vi "Query (varients).vi"(6 "timeout in ms (5000)":i32=5000, 8 "error in (no error)":errorcluster, 9 "Varient":variant, 10 "Label":string, 11 "MSR Parent":refnum<class "Send.lvclass">) -> (0 "error out":errorcluster, 1 "Replay Varient":variant, 2 "Reply Label":string, 3 "MSR Parent":refnum<class "Send.lvclass">)   [LabVIEW 2011, in "Messenging.lvlib" / "Send.lvclass"]
uses:
  Send.lvclass
  VarMessage/VarMessage.lvclass
  TextVarientMessage/MSG.lvclass
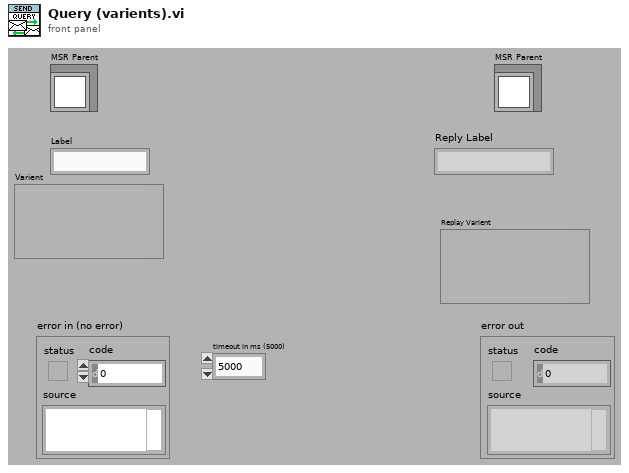
[diagram p1: front panel]
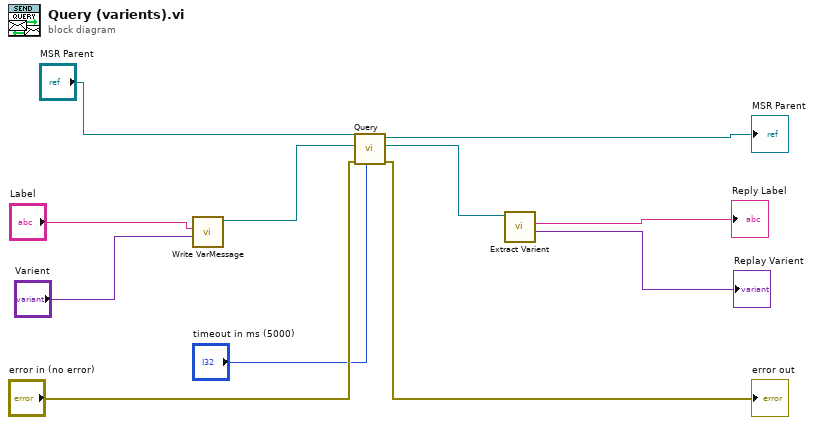
[diagram p0: block diagram]
diagram:
  n1 = call "Write VarMessage.vi"("Varient"="Varient", "Label"="Label") -> ("Message"=w2:refnum<class "VarMessage.lvclass">)  [unwired: 1 in, 8 out]
  n2 = call-dynamic "Query.vi"("timeout in ms (5000)"="timeout in ms (5000)", "error in (no error)"="error in (no error)", "Message"=w2, "MSR Parent"="MSR Parent") -> ("error out"=→"error out":errorcluster, "Reply"=w6:refnum<class "MSG.lvclass">, "MSR Parent"=→"MSR Parent":refnum<class "Send.lvclass">)  [unwired: 5 out]
  n3 = call-dynamic "Extract Varient.vi"("Message"=w6) -> ("Varient"=→"Replay Varient":variant, "Label"=→"Reply Label":string)  [unwired: 2 in, 7 out]
